vi "read_and_write_test.vi"() -> ()   [LabVIEW 2019]
uses:
  <vilib>/UPVI/lvhdf5/file.llb/LVH5F Operation.ctl
  <vilib>/Utility/miscctls.llb/LVRectTypeDef.ctl
  <vilib>/UPVI/lvhdf5/group.llb/H5G_obj_t.ctl
  <vilib>/UPVI/lvhdf5/dataset.llb/LVH5D Operation.ctl
  <vilib>/UPVI/lvhdf5/dataspace.llb/H5S_seloper_t.ctl
  <vilib>/UPVI/lvhdf5/utility.llb/Select HDF5 Dialog.vi
  <vilib>/UPVI/lvhdf5/utility.llb/Select HDF5 Dialog (Object Only).vi
  <vilib>/UPVI/lvhdf5/dataset.llb/Simple H5Dread (Variant).vi
  <vilib>/UPVI/lvhdf5/dataset.llb/Simple H5Dwrite (Variant).vi
  <vilib>/UPVI/lvhdf5/dataset.llb/H5Dwrite (Variant).vi
  <vilib>/UPVI/lvhdf5/dataset.llb/Simple H5Dread.xnode
  <vilib>/UPVI/lvhdf5/library.llb/HDF5 Ref.ctl
  <vilib>/UPVI/lvhdf5/dataset.llb/Simple H5Dwrite.xnode
  <vilib>/UPVI/lvhdf5/dataset.llb/H5Dwrite.xnode
  <vilib>/UPVI/lvhdf5/identifier.llb/Not an HDF5 Refnum Constant.vi
  <vilib>/Utility/error.llb/Error Cluster From Error Code.vi
  <vilib>/UPVI/lvhdf5/dataset.llb/OpenCreateReplace Dataset by Element Type.vi
  <vilib>/UPVI/lvhdf5/attribute.llb/private/LVH5AwriteWDTAttrs.vi
  <vilib>/UPVI/lvhdf5/dataspace.llb/H5Sclose.vi
  <vilib>/UPVI/lvhdf5/dataset.llb/H5Dclose.vi
  <vilib>/UPVI/lvhdf5/utility.llb/Select HDF5 Dialog (File and Object).vi
  <vilib>/UPVI/lvhdf5/file.llb/H5Fopen.vi
  <vilib>/UPVI/lvhdf5/dataset.llb/OpenCreateReplace Dataset.vi
  <vilib>/UPVI/lvhdf5/dataset.llb/H5Dread (Variant).vi
  <vilib>/UPVI/lvhdf5/attribute.llb/private/LVH5AreadWDTAttrs.vi
panel:
  in  "Text Ring":u16(ring) items=["Write", "Read", "Generate"]
  out "Count 2":i64
  out "Count":i64
  in  "Array 2":i32[][](array[numeric])
  out "Dims":u64[](array[numeric])
  out "Rank":i32
  out "Array":i32[][](array[numeric])
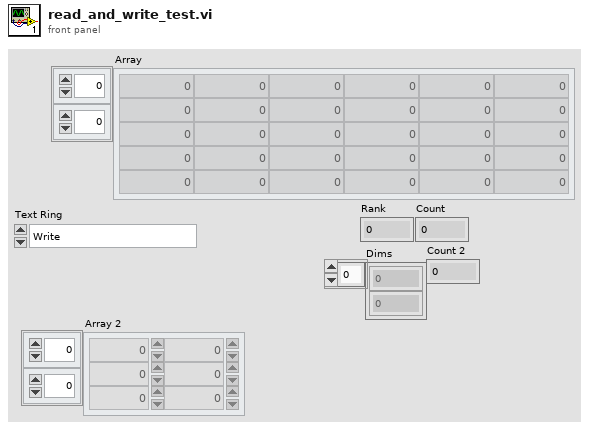
[diagram p1: front panel]
types:
  T1 = typedef "LVH5F Operation.ctl" = enum16{"open", "open or create", "create or replace", "create or replace (with confirmation)", "create", "open (read only)"}
  T2 = typedef "LVRectTypeDef.ctl" = cluster{"Left":i16, "Top":i16, "Right":i16, "Bottom":i16}
  T3 = cluster{"Behavior":enum32{"Invalid", "Default", "Floating", "Floating/Auto-Hide", "Modal"}, "Position":T2, "Center":bool, "Title":string}
  T4 = typedef "LVH5D Operation.ctl" = enum16{"open", "replace", "create", "open or create", "create or replace", "create or replace with confirmation"}
  T5 = typedef "H5G_obj_t.ctl" = i32
  T6 = cluster{"Object Types (any)":T5[], "Object Pattern":string}
  T7 = typedef "HDF5 Ref.ctl" = refnum<k1>
  T8 = typedef "H5S_seloper_t.ctl" = i32
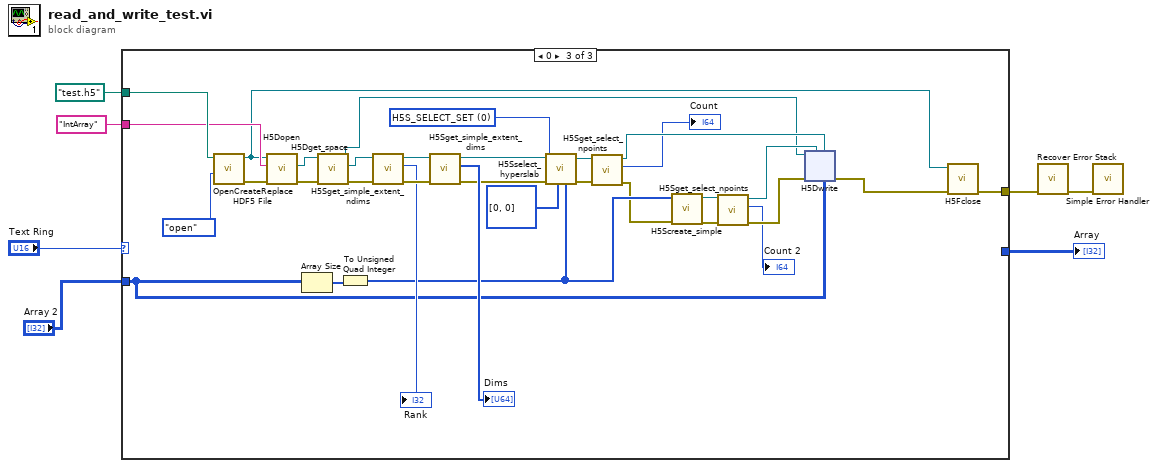
[diagram p0: block diagram]
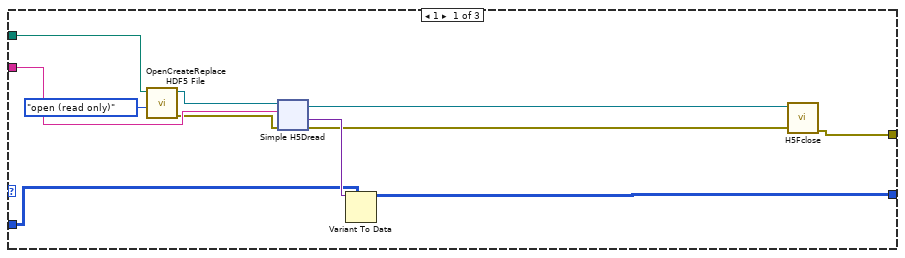
[diagram p2: hidden frame]
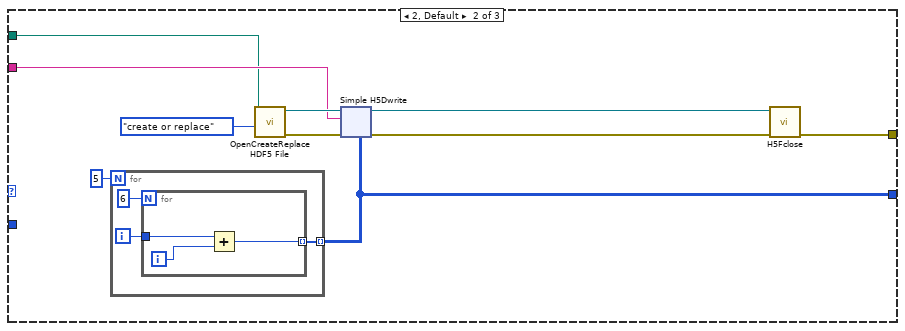
[diagram p3: hidden frame]
diagram:
  n1 = case shown="0" "Text Ring" {
    tunnel: "IntArray" ("Dataset Path") -> [w16 w341 w583]
    tunnel: path "test.h5" ("path") -> [w18 w339 w585]
    tunnel: [w14 w338 _] -> w5
    tunnel: [w12 w335 w576] -> w4
    tunnel: "Array 2" -> [w8 _ w553]
    frame 1 {
      n2 = call <vilib>:"OpenCreateReplace HDF5 File.vi"("function (open or create)"=LVH5F_Operation."open (read only)", "path"=w18) -> ("error out"=w11:errorcluster, "HDF5 Ref out"=w17:T7)  [unwired: 6 in]
      n3 = xnode "Simple H5Dread"("Dataset Path"=w16, "error in (no error)"=w11, "HDF5 Path or Ref"=w17) -> ("HDF5 Ref out"=w10:T7, "error out"=w13:errorcluster, "Data out"=w15:variant)  [unwired: 1 in, 1 out]
      n4 = Variant To Data(type=w8, Variant=w15) -> (data=w14:i32[][])  [unwired: 1 in, 1 out]
      n5 = call <vilib>:"H5Fclose.vi"("error in (no error)"=w13, "HDF5 Ref"=w10) -> ("error out"=w12:errorcluster)  [unwired: 7 in]
    }
    frame 2, Default {
      n6 = for {
        N: 5 -> [_]
        tunnel: [w345] -> w338 mode=indexing
        i -> [w346]
        n7 = for {
          N: 6 -> [_]
          tunnel: w346 -> [w350]
          tunnel: [w348] -> w345 mode=indexing
          i -> [w349]
          n8 = Add(x=w350, y=w349) -> (x+y=w348:i32)
        }
      }
      n9 = call <vilib>:"OpenCreateReplace HDF5 File.vi"("function (open or create)"=LVH5F_Operation."create or replace", "path"=w339) -> ("error out"=w342:errorcluster, "HDF5 Ref out"=w343:T7)  [unwired: 6 in]
      n10 = xnode "Simple H5Dwrite"("Dataset Path"=w341, "error in (no error)"=w342, "HDF5 Path or Ref"=w343, "Data"=w338) -> ("HDF5 Ref out"=w337:T7, "error out"=w336:errorcluster)  [unwired: 4 in, 1 out]
      n11 = call <vilib>:"H5Fclose.vi"("error in (no error)"=w336, "HDF5 Ref"=w337) -> ("error out"=w335:errorcluster)  [unwired: 7 in]
    }
    frame 0 {
      w571 = T8 0 items=["H5S_SELECT_NOOP"=-1, "H5S_SELECT_SET"=0, "H5S_SELECT_OR"=1, "H5S_SELECT_AND"=2, "H5S_SELECT_XOR"=3, "H5S_SELECT_NOTB"=4, "H5S_SELECT_NOTA"=5, "H5S_SELECT_APPEND"=6, "H5S_SELECT_PREPEND"=7] ("Operator")
      n12 = call <vilib>:"OpenCreateReplace HDF5 File.vi"("function (open or create)"=LVH5F_Operation."open", "path"=w585) -> ("error out"=w584:errorcluster, "HDF5 Ref out"=w568:T7)  [unwired: 6 in]
      n13 = call <vilib>:"H5Dopen.vi"("error in (no error)"=w584, "name"=w583, "HDF5 Ref"=w568) -> ("error out"=w582:errorcluster, "HDF5 Dataset Ref"=w579:T7)  [unwired: 4 in, 1 out]
      n14 = Array Size(array=w553) -> (size(s)=w567:i32[])
      n15 = call <vilib>:"H5Dget_space.vi"("error in (no error)"=w582, "HDF5 Dataset Ref"=w579) -> ("error out"=w581:errorcluster, "HDF5 Dataspace Ref"=w580:T7, "HDF5 Dataset Ref out"=w555:T7)  [unwired: 5 in]
      n16 = To Unsigned Quad Integer(1:w567) -> (0:w566:u64[])
      n17 = call <vilib>:"H5Sget_simple_extent_ndims.vi"("error in (no error)"=w581, "HDF5 Space Ref"=w580) -> ("error out"=w578:errorcluster, "Rank"=→"Rank":i32, "HDF5 Ref out"=w577:T7)  [unwired: 5 in]
      n18 = call <vilib>:"H5Sget_simple_extent_dims.vi"("error in (no error)"=w578, "HDF5 Space Ref"=w577) -> ("error out"=w573:errorcluster, "Dims"=→"Dims":u64[], "HDF5 Ref out"=w572:T7)  [unwired: 4 in, 1 out]
      n19 = call <vilib>:"H5Sselect_hyperslab.vi"("Count"=w566, "Start"=u64[] [0, 0], "error in (no error)"=w573, "Operator"=w571, "HDF5 Space Ref"=w572) -> ("error out"=w559:errorcluster, "HDF5 Ref out"=w561:T7)  [unwired: 5 in]
      n20 = call <vilib>:"H5Sget_select_npoints.vi"("error in (no error)"=w559, "HDF5 Space Ref"=w561) -> ("error out"=w558:errorcluster, "Count"=→"Count":i64, "HDF5 Ref out"=w560:T7)  [unwired: 5 in]
      n21 = call <vilib>:"H5Screate_simple.vi"("error in (no error)"=w558, "Dimensions"=w566) -> ("error out"=w565:errorcluster, "HDF5 Ref out"=w563:T7)  [unwired: 6 in]
      n22 = call <vilib>:"H5Sget_select_npoints.vi"("error in (no error)"=w565, "HDF5 Space Ref"=w563) -> ("error out"=w564:errorcluster, "Count"=→"Count 2":i64, "HDF5 Ref out"=w562:T7)  [unwired: 5 in]
      n23 = xnode "H5Dwrite"("HDF5 Dataset Ref"=w555, "HDF5 File Space Ref (H5S_ALL)"=w560, "HDF5 Memory Space Ref (H5S_ALL)"=w562, "error in (no error)"=w564, "Data"=w553) -> ("error out"=w569:errorcluster)  [unwired: 2 in, 1 out]
      n24 = call <vilib>:"H5Fclose.vi"("error in (no error)"=w569, "HDF5 Ref"=w568) -> ("error out"=w576:errorcluster)  [unwired: 7 in]
    }
  }
  "Array" <- w5
  n25 = call <vilib>:"Recover Error Stack.vi"("error in (no error)"=w4) -> ("error out"=w3:errorcluster)  [unwired: 5 in, 3 out]
  n26 = call <vilib>:"Simple Error Handler.vi"("error in (no error)"=w3) -> ()  [unwired: 4 in, 5 out]
